vi "SearchNextEmptyCell.vi"(11 "Board":i32[][](array[numeric])) -> (0 "empty Cell found?":bool, 1 "Cell":T1, 3 "Board":i32[][](array[numeric]))   [LabVIEW 2023]
doc: "In current Board, search for next emply cell in and return its row and colum\n\nInputs\n- Board: Current Board Configuration\n\nOutputs\n- Board: Current Board Configuration\n- Row: Row of next empty Cell\n- Column: Column of next empty Cell"
uses:
  Controls/CurrentCell.ctl
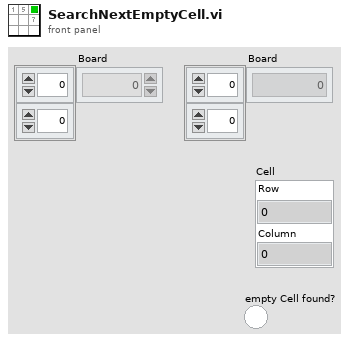
[diagram p1: front panel]
types:
  T1 = typedef "CurrentCell.ctl" = cluster{"Row":i32, "Column":i32}
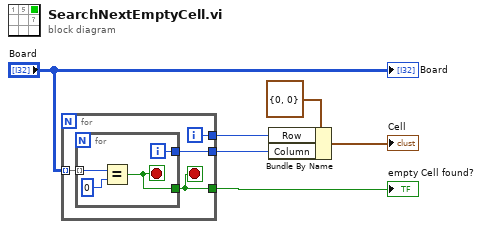
[diagram p0: block diagram]
diagram:
  n1 = for {
    tunnel: "Board" -> [w10] mode=indexing
    tunnel: [w9] -> w3
    tunnel: [w8] -> w2
    tunnel: [w7] -> w5
    i -> [w9]
    stop <- w7 stop-if-true
    n2 = for {
      tunnel: w10 -> [w14] mode=indexing
      tunnel: [w12] -> w7
      tunnel: [w11] -> w8
      i -> [w11]
      stop <- w12 stop-if-true
      n3 = Equal?(x=w14, y=0) -> (x = y?=w12:bool)
    }
  }
  "empty Cell found?" <- w5
  n4 = Bundle By Name(cluster=T1 {"Row"=0, "Column"=0} ("Current Cell"), "Row"=w3, "Column"=w2) -> (→"Cell":T1)
  "Board" <- "Board"
